vi "PipBoy_ProcPipComm.vi"(8 "error in (no error)":errorcluster, 10 "PipBoyData":T1) -> (0 "error out":errorcluster)   [LabVIEW 2014]
uses:
  ctls/PipBoy_PipBoyData.ctl
  ctls/PipBoy_ProcComm.ctl
  System.Windows.Forms
  ctls/PipBoy_PipBoyCommand.ctl
  ctls/PipBoy_Message.ctl
  modules/support/Message Queue/All Message Queues.ctl
  modules/support/Message Queue/Message Cluster.ctl
  ctls/PipBoy_FileConf.ctl
  ctls/PipBoy_PicComm.ctl
  ctls/PipBoy_GeneralParams.ctl
  ctls/PipBoy_Pages.ctl
  <vilib>/Instr/_visa.llb/VISA Open Access Mode.ctl
  <vilib>/Utility/error.llb/Error Cluster From Error Code.vi
  <vilib>/ErrorRing/Error Ring.xnode
  modules/support/Message Queue/Message Queue.lvlib
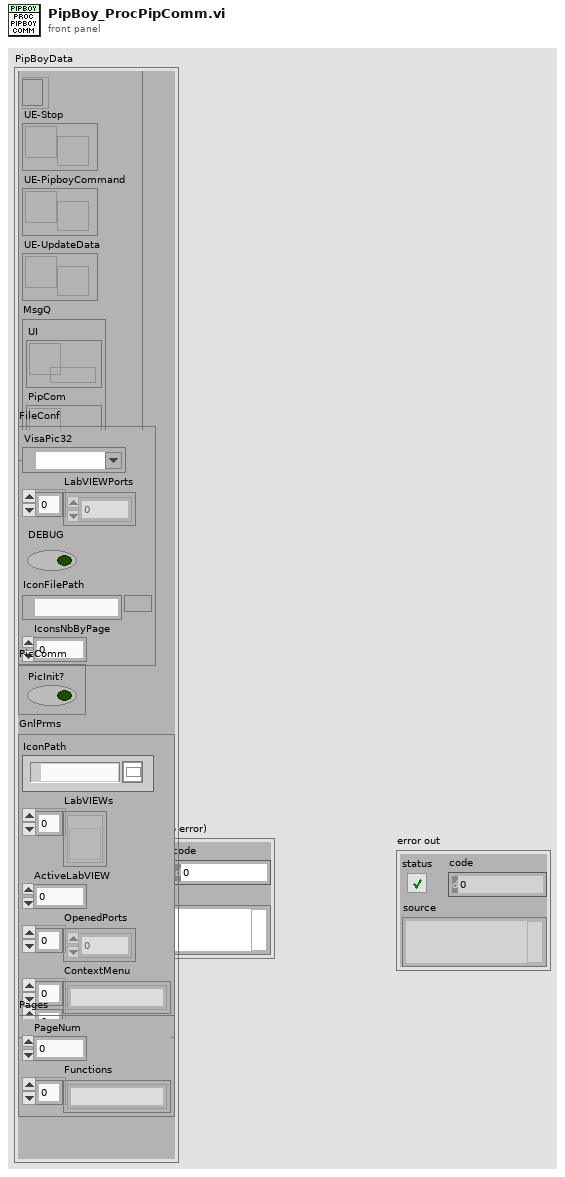
[diagram p1: front panel]
types:
  T1 = typedef "PipBoy_PipBoyData.ctl" = cluster{"ProcComm":T2, "FileConf":T4, "PicComm":T5, "GnlPrms":T6, "Pages":T7}
  T2 = typedef "PipBoy_ProcComm.ctl" = cluster{"NotifyIconRef":refnum<k24>, "UE-Stop":refnum<user-event>, "UE-PipboyCommand":refnum<user-event>, "UE-UpdateData":refnum<user-event>, "MsgQ":T3}
  T3 = typedef "Message Queue.lvlib/All Message Queues.ctl" = cluster{"UI":refnum<queue>, "PipCom":refnum<queue>}
  T4 = typedef "PipBoy_FileConf.ctl" = cluster{"VisaPic32":refnum<visa-resource-name>, "LabVIEWPorts":u16[], "DEBUG":bool, "IconFilePath":path, "IconsNbByPage":i32}
  T5 = typedef "PipBoy_PicComm.ctl" = cluster{"PicInit?":bool}
  T6 = typedef "PipBoy_GeneralParams.ctl" = cluster{"IconPath":path, "LabVIEWs":refnum<vi>[], "ActiveLabVIEW":i32, "OpenedPorts":u16[], "ContextMenu":string[][]}
  T7 = typedef "PipBoy_Pages.ctl" = cluster{"PageNum":i32, "Functions":string[]}
  T8 = typedef "VISA Open Access Mode.ctl" = u32
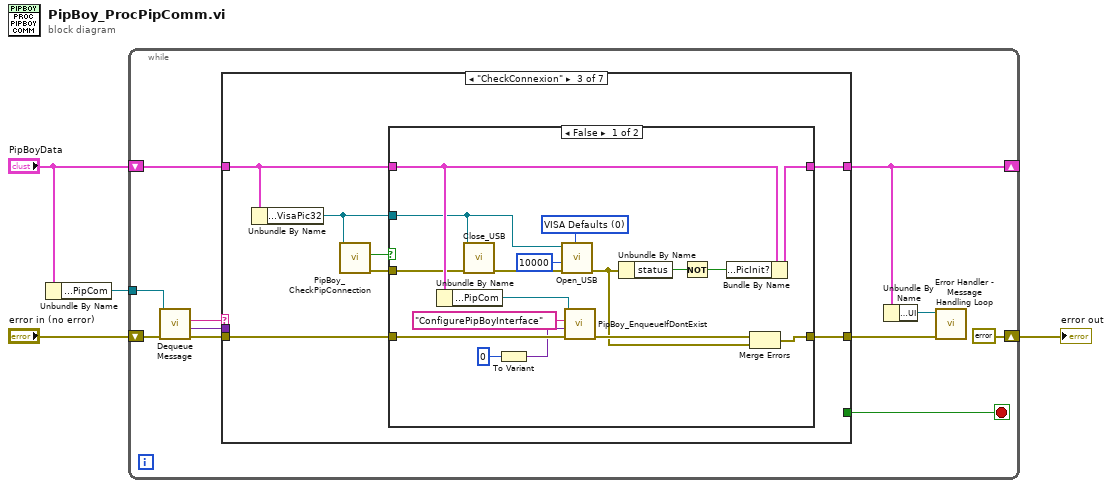
[diagram p0: block diagram]
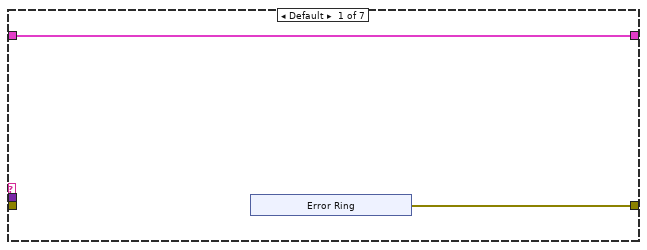
[diagram p2: hidden frame]
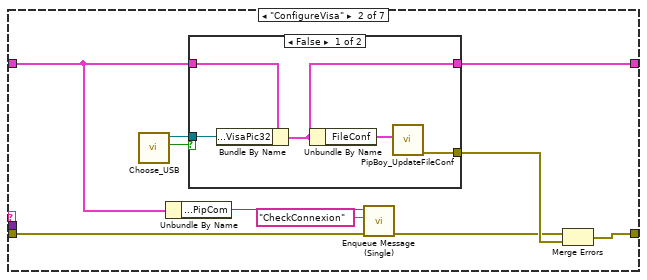
[diagram p3: hidden frame]
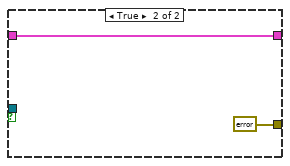
[diagram p4: hidden frame]
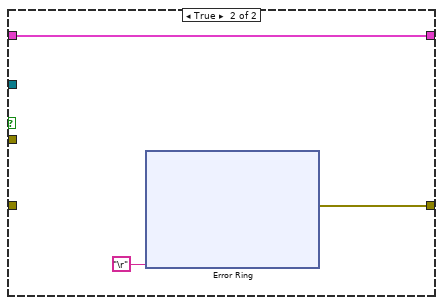
[diagram p5: hidden frame]
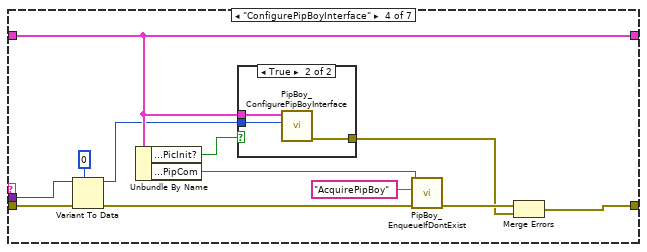
[diagram p6: hidden frame]
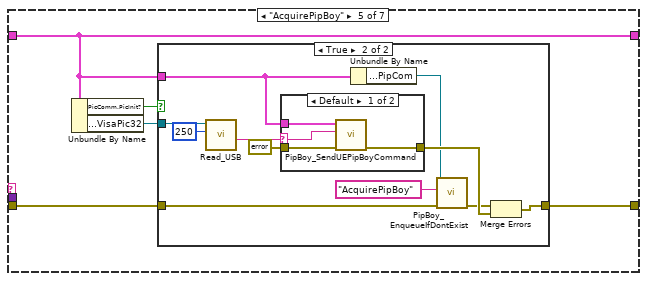
[diagram p8: hidden frame]
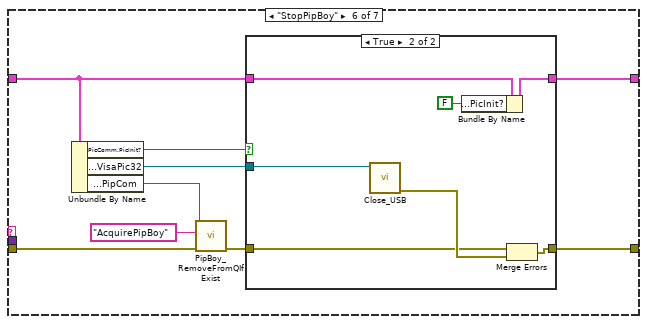
[diagram p11: hidden frame]
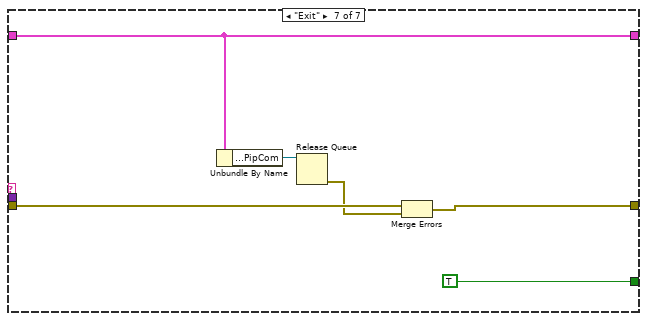
[diagram p13: hidden frame]
diagram:
  n1 = Unbundle By Name("PipBoyData") -> ("ProcComm.MsgQ.PipCom"=w1:refnum<queue>)
  n2 = while {
    shift-right: [errorcluster {"status"=FALSE, "code"=0, "source"=""} ("error in (no error)")] -> w3
    shift-left: "error in (no error)" -> [w12]
    shift-right: [w9] -> _
    shift-left: "PipBoyData" -> [w10]
    tunnel: w1 -> [w7]
    stop <- w13 stop-if-true
    n3 = call "Dequeue Message.vi"("error in (no error)"=w12, "Message Queue"=w7) -> ("error out"=w11:errorcluster, "Message Data"=w5:variant, "Message"=w15:string)  [unwired: 6 in, 1 out]
    n4 = case shown="\"CheckConnexion\"" w15 {
      tunnel: [w16 w32 w45 w84 w92 w117 w134] -> w14
      tunnel: [_ _ _ _ _ _ TRUE] -> w13
      tunnel: w11 -> [_ w26 w46 w78 w93 w114 w131]
      tunnel: w10 -> [w17 w24 w42 w80 w89 w116 w129]
      tunnel: [w17 w30 w44 w80 w89 w115 w129] -> w9
      tunnel: w5 -> [_ _ _ w76 _ _ _]
      frame Default {
        n5 = xnode "Error Ring"() -> ("error out"=w16:errorcluster)
      }
      frame "ConfigureVisa" {
        n6 = call "Choose_USB.vi"() -> ("Annulé?"=w31:bool, "Nom de ressource VISA en sortie"=w29:refnum<visa-resource-name>)  [unwired: 10 in]
        n7 = Unbundle By Name(w24) -> ("ProcComm.MsgQ.PipCom"=w23:refnum<queue>)
        n8 = case shown="False" w31 {
          tunnel: [w33 w39] -> w30
          tunnel: w24 -> [w37 w39]
          tunnel: w29 -> [w34 _]
          tunnel: [w36 errorcluster {"status"=FALSE, "code"=0, "source"=""} ("error out")] -> w28
          frame False {
            n9 = Bundle By Name(cluster=w37, "FileConf.VisaPic32"=w34) -> (w33:T1)
            n10 = Unbundle By Name(w33) -> ("FileConf"=w35:T4)
            n11 = call "PipBoy_UpdateFileConf.vi"("FileConf"=w35) -> ("error out"=w36:errorcluster)  [unwired: 10 in]
          }
          frame True {
          }
        }
        n12 = call "Enqueue Message (Single).vi"("error in (no error)"=w26, "Message"="CheckConnexion", "Message Queue"=w23) -> ("error out"=w25:errorcluster)  [unwired: 7 in, 1 out]
        n13 = Merge Errors(w25, w28) -> (w32:errorcluster)
      }
      frame "CheckConnexion" {
        n14 = Unbundle By Name(w42) -> ("FileConf.VisaPic32"=w41:refnum<visa-resource-name>)
        n15 = call "PipBoy_CheckPipConnection.vi"("VISAPic32"=w41) -> ("error out"=w43:errorcluster, "Error ?"=w40:bool)  [unwired: 9 in]
        n16 = case shown="False" w40 {
          tunnel: w42 -> [w57 w66]
          tunnel: [w63 w66] -> w44
          tunnel: w46 -> [w59 _]
          tunnel: [w60 w65] -> w45
          tunnel: w43 -> [w48 _]
          tunnel: w41 -> [w49 _]
          frame False {
            w61 = T8 0 items=["VISA Defaults"=0, "Exclusive Lock"=1, "Load Configured Settings"=4] ("Access Mode")
            n17 = Unbundle By Name(w57) -> ("ProcComm.MsgQ.PipCom"=w52:refnum<queue>)
            n18 = call "Close_USB.vi"("entrée d'erreur"=w48, "Nom de ressource VISA"=w49) -> ("sortie d'erreur"=w47:errorcluster)  [unwired: 9 in]
            n19 = To Variant(anything=0 ("Pages.PageNum")) -> (Variant=w50:variant)
            n20 = call "Open_USB.vi"("entrée d'erreur"=w47, "Timeout (100)"=u32 10000 ("Timeout de VISA Open (0)"), "Access Mode"=w61, "Nom de ressource VISA"=w49) -> ("error out"=w56:errorcluster)  [unwired: 6 in, 1 out]
            n21 = call "PipBoy_EnqueueIfDontExist.vi"("error in (no error)"=w59, "Message Data"=w50, "Message"="ConfigurePipBoyInterface", "Message Queue"=w52) -> ("error out"=w58:errorcluster)  [unwired: 7 in]
            n22 = Unbundle By Name(w56) -> ("status"=w55:bool)
            n23 = Not(x=w55) -> (.not. x?=w54:bool)
            n24 = Bundle By Name(cluster=w57, "PicComm.PicInit?"=w54) -> (w63:T1)
            n25 = Merge Errors(w58, w56) -> (w60:errorcluster)
          }
          frame True {
            n26 = xnode "Error Ring"("parameter 0"="\r") -> ("error out"=w65:errorcluster)
          }
        }
      }
      frame "ConfigurePipBoyInterface" {
        n27 = Variant To Data(error in=w78, type=0 ("PageNum"), Variant=w76) -> (data=w74:i32, error out=w77:errorcluster)
        n28 = Unbundle By Name(w80) -> ("PicComm.PicInit?"=w81:bool, "ProcComm.MsgQ.PipCom"=w79:refnum<queue>)
        n29 = case shown="True" w81 {
          tunnel: [_ w88] -> w83
          tunnel: w80 -> [_ w87]
          tunnel: w74 -> [_ w86]
          frame False {
          }
          frame True {
            n30 = call "PipBoy_ConfigurePipBoyInterface.vi"("PageNum"=w86, "PipBoyData"=w87) -> ("error out"=w88:errorcluster)  [unwired: 9 in]
          }
        }
        n31 = call "PipBoy_EnqueueIfDontExist.vi"("error in (no error)"=w77, "Message"="AcquirePipBoy", "Message Queue"=w79) -> ("error out"=w85:errorcluster)  [unwired: 8 in]
        n32 = Merge Errors(w85, w83) -> (w84:errorcluster)
      }
      frame "AcquirePipBoy" {
        n33 = Unbundle By Name(w89) -> ("PicComm.PicInit?"=w90:bool, "FileConf.VisaPic32"=w91:refnum<visa-resource-name>)
        n34 = case shown="True" w90 {
          tunnel: w93 -> [w94 w100]
          tunnel: [w94 w105] -> w92
          tunnel: w91 -> [_ w104]
          tunnel: w89 -> [_ w95]
          frame False {
          }
          frame True {
            n35 = call "Read_USB.vi"("timeout (0)"=u32 250, "Nom de ressource VISA"=w104) -> ("chaîne en sortie"=w103:string)  [unwired: 7 in, 2 out]
            n36 = case shown="Default" w103 {
              selector: w103 -> [w107 _]
              tunnel: [w108 w110] -> w102
              tunnel: errorcluster {"status"=FALSE, "code"=0, "source"=""} ("sortie d'erreur") -> [w109 w110]
              tunnel: w95 -> [w106 _]
              frame Default {
                n37 = call "PipBoy_SendUEPipBoyCommand.vi"("error in (no error)"=w109, "Command"=w107, "PipBoyData"=w106) -> ("error out"=w108:errorcluster)  [unwired: 8 in]
              }
              frame "" {
              }
            }
            n38 = Unbundle By Name(w95) -> ("ProcComm.MsgQ.PipCom"=w101:refnum<queue>)
            n39 = call "PipBoy_EnqueueIfDontExist.vi"("error in (no error)"=w100, "Message"="AcquirePipBoy", "Message Queue"=w101) -> ("error out"=w99:errorcluster)  [unwired: 8 in]
            n40 = Merge Errors(w99, w102) -> (w105:errorcluster)
          }
        }
      }
      frame "StopPipBoy" {
        n41 = Unbundle By Name(w116) -> ("PicComm.PicInit?"=w119:bool, "FileConf.VisaPic32"=w118:refnum<visa-resource-name>, "ProcComm.MsgQ.PipCom"=w111:refnum<queue>)
        n42 = call "PipBoy_RemoveFromQIfExist.vi"("error in (no error)"=w114, "Message"="AcquirePipBoy", "Message Queue"=w111) -> ("error out"=w113:errorcluster)  [unwired: 8 in]
        n43 = case shown="True" w119 {
          tunnel: w113 -> [w121 w122]
          tunnel: [w121 w128] -> w117
          tunnel: w118 -> [_ w127]
          tunnel: w116 -> [w120 w124]
          tunnel: [w120 w123] -> w115
          frame False {
          }
          frame True {
            n44 = call "Close_USB.vi"("Nom de ressource VISA"=w127) -> ("sortie d'erreur"=w126:errorcluster)  [unwired: 10 in]
            n45 = Bundle By Name(cluster=w124, "PicComm.PicInit?"=FALSE) -> (w123:T1)
            n46 = Merge Errors(w122, w126) -> (w128:errorcluster)
          }
        }
      }
      frame "Exit" {
        n47 = Unbundle By Name(w129) -> ("ProcComm.MsgQ.PipCom"=w132:refnum<queue>)
        n48 = Release Queue(queue=w132) -> (error out=w130:errorcluster)  [unwired: 2 in, 2 out]
        n49 = Merge Errors(w131, w130) -> (w134:errorcluster)
      }
    }
    n50 = Unbundle By Name(w9) -> ("ProcComm.MsgQ.UI"=w8:refnum<queue>)
    n51 = call "Error Handler - Message Handling Loop.vi"("error in (no error)"=w14, "Message Queue"=w8) -> ()  [unwired: 8 in, 2 out]
  }
  "error out" <- w3
